vi "Schedule Job.vi"(4 "Start Time":i32, 5 "fInsert":bool, 6 "Processing Times":u16[][](array[numeric]), 7 "Operation":i32, 8 "Index to schedule/Insert":i32, 9 "Job Number":i32, 10 "Machine No":i32, 11 "Gannt Chart In":T1[][](array[typedef])) -> (3 "Gannt Chart Out":T1[][](array[typedef]))   [LabVIEW 2013, in "Scheduler.lvclass"]
uses:
  Scheduler.lvclass
  Controls/GanntChart_Element.ctl
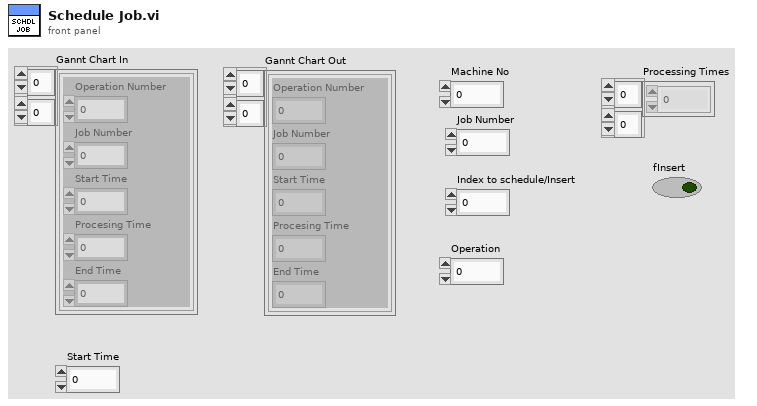
[diagram p1: front panel]
types:
  T1 = typedef "GanntChart_Element.ctl" = cluster{"Operation Number":i32, "Job Number":i32, "Start Time":i32, "Procesing Time":u16, "End Time":i32}
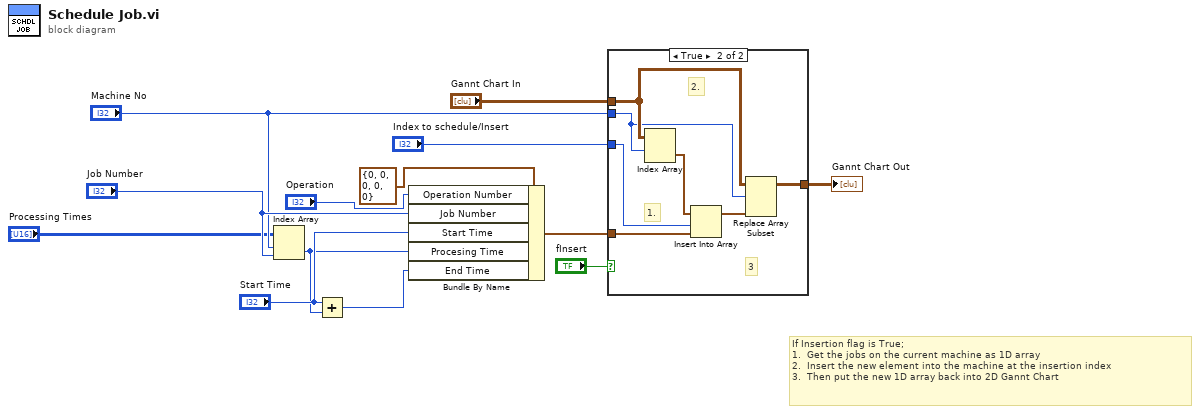
[diagram p0: block diagram]
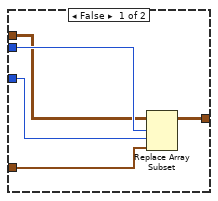
[diagram p2: hidden frame]
diagram:
  # "If Insertion flag is True;\n1.  Get the jobs on the current machine as 1D array\n2.  Insert the new element into the machine at the insertion index\n3.  Then put the new 1D array back into 2D Gannt Chart"
  n1 = Index Array(array="Processing Times", index (row)="Machine No", index (col)="Job Number") -> (element=w3:u16)
  n2 = Add(x="Start Time", y=w3) -> (x+y=w2:i32)
  n3 = Bundle By Name(cluster=T1 {"Operation Number"=0, "Job Number"=0, "Start Time"=0, "Procesing Time"=0, "End Time"=0} ("new element/subarray"), "Operation Number"="Operation", "Job Number"="Job Number", "Start Time"="Start Time", "Procesing Time"=w3, "End Time"=w2) -> (w5:T1)
  n4 = case shown="True" "fInsert" {
    tunnel: [w18 w19] -> w13
    tunnel: "Machine No" -> [w17 w21]
    tunnel: "Index to schedule/Insert" -> [w16 w24]
    tunnel: "Gannt Chart In" -> [w15 w22]
    tunnel: w5 -> [w14 w23]
    frame False {
      n5 = Replace Array Subset(array=w15, new element=w14, index (row)=w17, index (col)=w16) -> (w18:T1[][])
    }
    frame True {
      # "3"
      # "2."
      # "1."
      n6 = Index Array(array=w22, index (row)=w21) -> (element=w25:T1[])  [unwired: 1 in]
      n7 = Insert Into Array(array=w25, index=w24, new element=w23) -> (w20:T1[])
      n8 = Replace Array Subset(array=w22, new element=w20, index (row)=w21) -> (w19:T1[][])  [unwired: 1 in]
    }
  }
  "Gannt Chart Out" <- w13
